vi "LSX Get Switch Type.vi"(0 "lLSID":i32, 1 "plRP":i32, 5 "plXP":i32, 7 "plYP":i32, 9 "plZP":i32, 11 "error in (no error)":errorcluster) -> (3 "plRP out":i32, 4 "function return":i32, 6 "plXP out":i32, 8 "plYP out":i32, 10 "plZP out":i32, 15 "error out":errorcluster)   [LabVIEW 2018, in "Tango.lvlib"]
doc: "TANGOAPI int TANGOCALL LSX_GetSwitchType (int lLSID, int *plXP, int *plYP, int *plZP, int *plRP);"
uses:
  Tango.lvlib
  SubVIs/Tango_DLL.dll
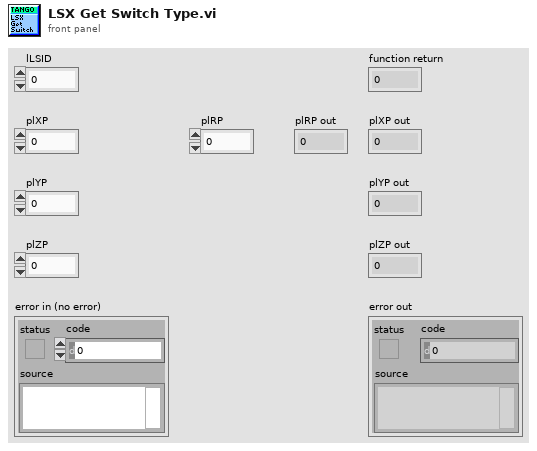
[diagram p1: front panel]
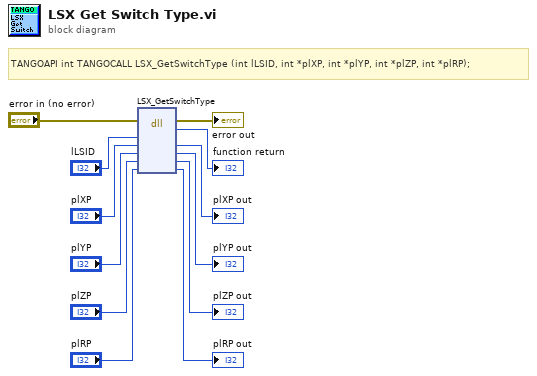
[diagram p0: block diagram]
diagram:
  # "TANGOAPI int TANGOCALL LSX_GetSwitchType (int lLSID, int *plXP, int *plYP, int *plZP, int *plRP);"
  n1 = dll-call lib="C:/Users/Familie/Documents/LabviewIX81/lib/TANGO Stage/SubVIs/Tango_DLL.*" fn="LSX_GetSwitchType"(error in="error in (no error)", "lLSID"="lLSID", "plXP"="plXP", "plYP"="plYP", "plZP"="plZP", "plRP"="plRP") -> (error out=→"error out":errorcluster, →"function return":i32, "plXP"=→"plXP out":i32, "plYP"=→"plYP out":i32, "plZP"=→"plZP out":i32, "plRP"=→"plRP out":i32)  [unwired: 3 in, 1 out]
